vi "Stop Core.vi"(10 "final error code":i32, 11 "LHW-Aquisition-Actor in":refnum<class "LHW-Aquisition-Actor.lvclass">) -> (3 "LHW-Aquisition-Actor out":refnum<class "LHW-Aquisition-Actor.lvclass">)   [LabVIEW 2016, in "LHW-Acquisition.lvlib" / "LHW-Aquisition-Actor.lvclass"]
doc: "(<B>Filename</B>: Actor Framework.lvlib:Actor.lvclass:Stop Core.vi)\n\nDefines what the actor does before it stops. Use the <B>final error code</B> input to determine whether the actor shut down in response to an error.\n\nBy default, this method does nothing. A descendant class may override it to define behavior, such as shutting down any processes the actor initiated in its override of the Actor Core method."
uses:
  LHW-Aquisition-Actor.lvclass
  <vilib>/ActorFramework/Actor/Actor.lvclass
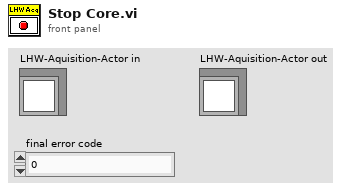
[diagram p1: front panel]
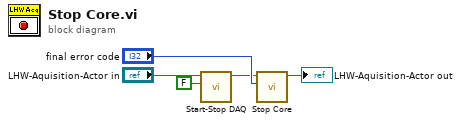
[diagram p0: block diagram]
diagram:
  n1 = call "Start-Stop DAQ.vi"("Start DAQ"=FALSE, "LHW-Aquisition-Actor in"="LHW-Aquisition-Actor in") -> ("LHW-Aquisition-Actor out"=w2:refnum<class "LHW-Aquisition-Actor.lvclass">)  [unwired: 8 in, 1 out]
  n2 = call-parent "Stop Core.vi"("final error code"="final error code", "Actor in"=w2) -> ("Actor out"=→"LHW-Aquisition-Actor out":refnum<class "LHW-Aquisition-Actor.lvclass">)  [unwired: 9 in]
